vi "Motion Profile Tester.vi"() -> ()   [LabVIEW 2015]
uses:
  <vilib>/Rock Robotics/WPI/CAN/TalonSRX/WPI_CANTalonSRX_APIFeedbackSelect.ctl
  <vilib>/Rock Robotics/WPI/CAN/TalonSRX/WPI_CANTalonSRX_MotionProfileTrajectoryPt.ctl
  <vilib>/Rock Robotics/WPI/CAN/TalonSRX/WPI_CANTalonSRX_APIControlMode.ctl
  <vilib>/Rock Robotics/WPI/MotorControl/WPI_MotorControlOpenCANTalonSRX.vi
panel:
  in  "Finish":bool
  in  "(Native Position units/sec)/(Native units for velocity)":dbl
  in  "Quantity of Points to Load Initially":dbl=126.0
  out "Loaded Trajectory Points":u32
  in  "Slave Motor Inverts":bool[](array[boolean])
  in  "Motor ID":dbl
  in  "Slave Motor IDs":dbl[](array[numeric])
  out "Current State":T1(ring)
  in  "Invert Motor":bool=TRUE
  in  "Execute Motion Profile using only Feedfoward":bool
  in  "Soft Limits (rotations)":T2={"Forward Limit Position"=10000.0, "Reverse Limit Position (should be less than foward limit position)"=-10000.0}
  in  "Reverse Soft Limit Enable":bool
  in  "Forward Soft Limit Enable":bool
  in  "Reverse Feedback Sensor":bool
  in  "Feedback Reference":T3=enum."CTR Magnetic Enc (Absolute)"
  in  "PID Values":T4={"P"=0.21, "I"=0.0021, "D"=3.0, "F"=0.12, "I Zone"=1200.0}
  out "error out":errorcluster
  out "Motor Values while Running Profile":cluster{dbl[], dbl[]}[](graph)
  out "Applied Throttle while Running Profile":cluster{dbl[], dbl[]}(graph)
  in  "Run at 100% Power and Graph":bool
  in  "Abort":bool
  in  "Generate, Load, and Run Profile":bool
  in  "Run Profile":bool
  in  "Load Profile":bool
  in  "Generate Profile and Clear Points":bool
  out "Generated Profile":cluster{dbl[], dbl[]}[](graph)
  in  "Mode":T1(ring)
  in  "Duration MS":dbl=10.0
  in  "Rotations to Travel":dbl
  in  "Max Jerk (rotations/sec^3)":dbl
  in  "Max Acceleration (rotations/sec^2)":dbl
  in  "Max Speed (rotations/sec)":dbl
  # "Basic Motor Configuration Settings"
  # "Motion Profile Settings"
  # "If applied throttle exceeds about .95 consistantly in the execution of the profile either max speed acceleration, or jerk must be lowered (or PIDF should be adjusted). If it goes below .8 except at the very beginning or end either max speed, acceleration, or jerk  could be increased. (These numbers are for profiles which are supposed to be completed as quickly as possible. In contexts where the priority is on other things such as reducing the amount of force or jerk acting on a gearbox other metrics must be used.)"
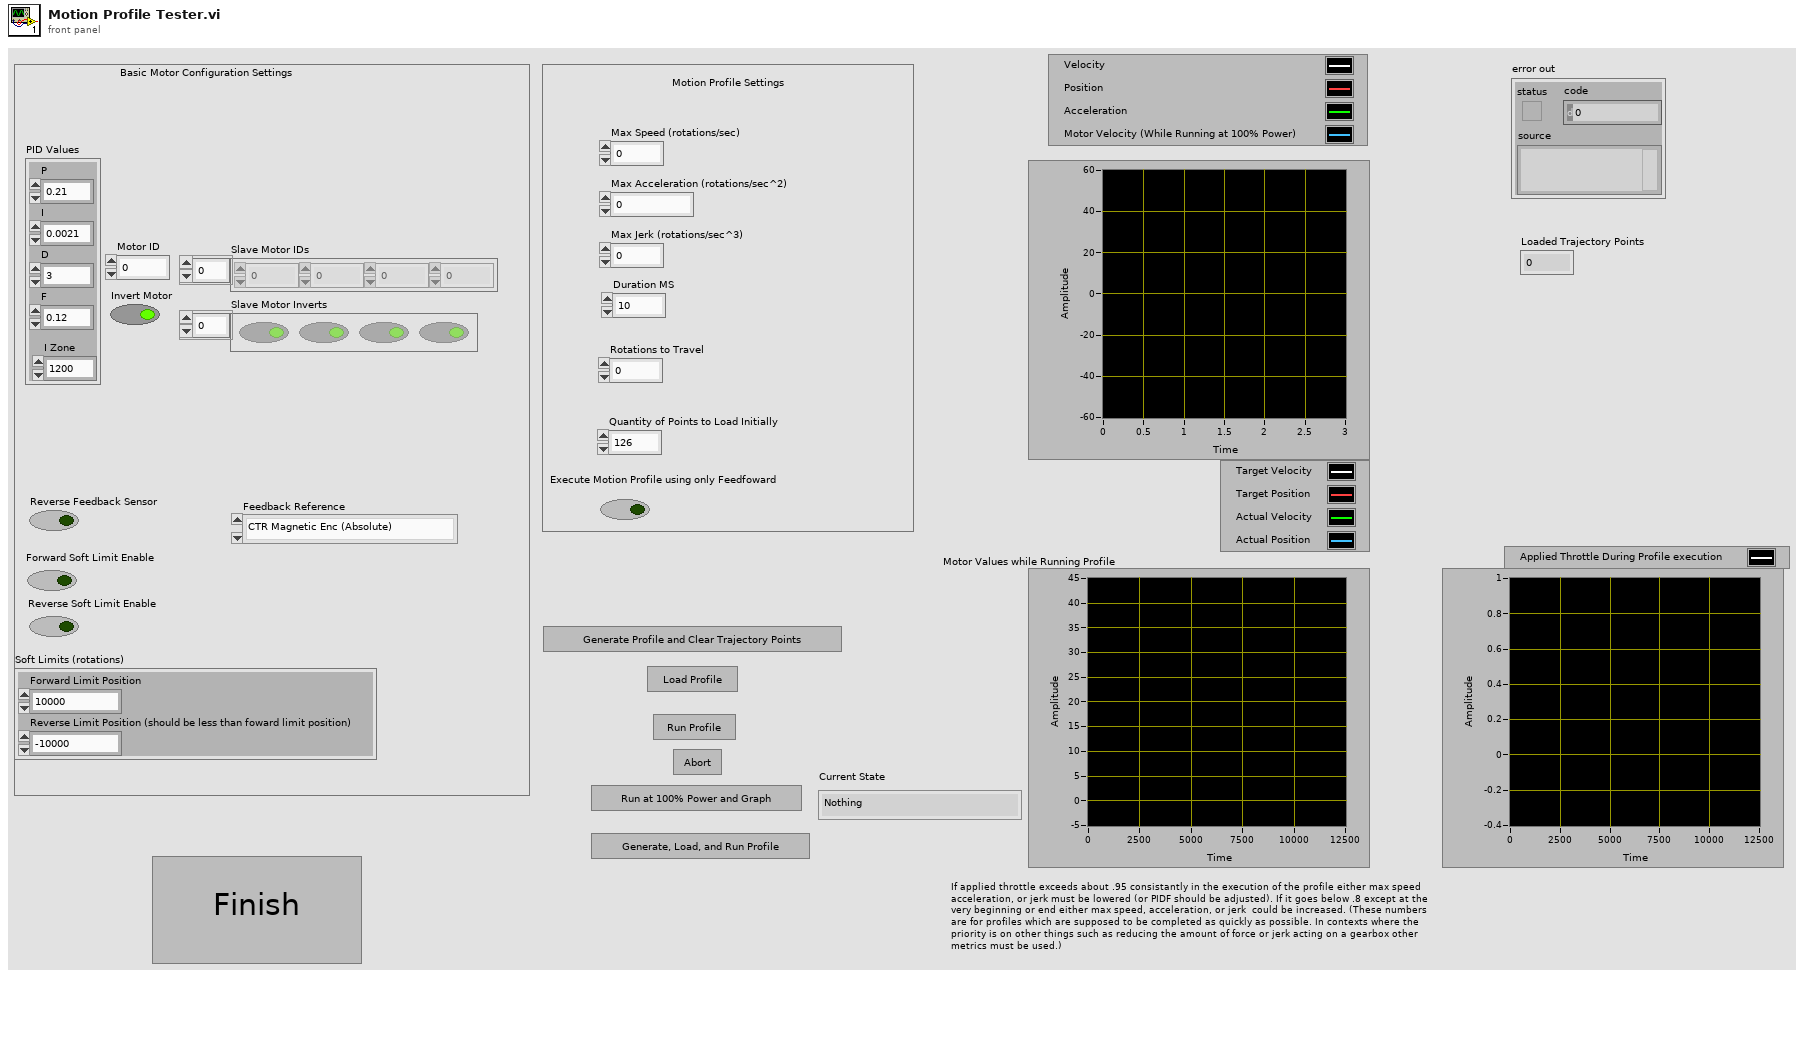
[diagram p1: front panel]
types:
  T1 = enum16{"Nothing", "Generate Profile and Clear", "Load Data to Motor", "Run Profile", "Run at 100% power and log"}
  T2 = cluster{"Forward Limit Position":dbl, "Reverse Limit Position (should be less than foward limit position)":dbl}
  T3 = typedef "WPI_CANTalonSRX_APIFeedbackSelect.ctl" = enum16{"Digital Quadrature Encoder", "Analog Potentiometer", "Analog Encoder", "Count on Quad-A (Rising-Edge)", "Count on Quad-A (Falling-Edge)", "CTR Magnetic Enc (Absolute)", "CTR Magnetic Enc (Relative)", "Pulse Width"}
  T4 = cluster{"P":dbl, "I":dbl, "D":dbl, "F":dbl, "I Zone":dbl}
  T5 = typedef "WPI_CANTalonSRX_APIControlMode.ctl" = enum8{"Percent VBus", "Speed", "Position", "Slave", "Unchanged / Invalid", "Voltage Compensation", "Current", "Motion Profile"}
  T6 = typedef "WPI_MotorControlDeviceRef.ctl" = cluster{"DeviceStatus":errorcluster, "Type":T7, "PWM":cluster{"PWM Channel":T8, "DeadBand":T9}, "CAN":cluster{"Device Number":u8, "Control Mode":T10, "Semaphore":T11, "Max Vout":dbl, "TalonSRX Control Mode":T5}, "Invert":bool}
  T7 = typedef "WPI_MotorControlType.ctl" = enum16{"PWM", "CAN", "CANTalonSRX"}
  T8 = typedef "FPGA_DIOPWMChannel.ctl" = enum8{"PWM 0", "PWM 1", "PWM 2", "PWM 3", "PWM 4", "PWM 5", "PWM 6", "PWM 7", "PWM 8", "PWM 9", "PWM MXP 0", "PWM MXP 1", "PWM MXP 2", "PWM MXP 3", "PWM MXP 4", "PWM MXP 5", "PWM MXP 6", "PWM MXP 7", "PWM MXP 8", "PWM MXP 9", "Invalid"}
  T9 = typedef "WPI_PWMDeadband.ctl" = cluster{"Name":string, "maxPositivePwm":i32, "minPositivePwm":i32, "centerPwm":i32, "maxNegativePwm":i32, "minNegativePwm":i32, "angularRange":u16}
  T10 = typedef "WPI_CANJaguar_ControlMode.ctl" = enum8{"Percent VBus", "Current", "Speed", "Position", "Voltage"}
  T11 = typedef "Semaphore RefNum" = refnum<k1>
  T12 = typedef "WPI_CANTalonSRX_MotionProfileTrajectoryPt.ctl" = cluster{"Duration Ms":u8, "Velocity":dbl, "Position":dbl, "Profile Slot Select":u8, "Is Last":bool, "Velocity Only":bool, "Zero Position":bool, "Compress Code":u8, "Same Velocity":i32, "Delta Position":i32, "Count":u8}
  T13 = enum16{"Nothing", "Generate Profile and Clear", "Load Data to Motor", "Run Profile"}
  T14 = enum16{"Nothing", "Generate Profile and Clear", "Load Data to Motor", "Run Profile", "Run at 100% power and log"}[]
  T15 = typedef "WPI_CANTalonSRX_GlobalStatus.ctl" = cluster{"Applied Throttle":dbl, "Module Enabled":bool, "CAN Error":errorcluster, "Closed Loop Error":dbl, "Forward Limit Switch Closed":bool, "Reverse Limit Switch Closed":bool, "Sensor Position":dbl, "Sensor Velocity":dbl, "Current":dbl, "Sticky Fault - Over Temp":bool, "Sticky Fault - Under Voltage":bool, "Sticky Fault - Forward Limit":bool, "Sticky Fault - Reverse Limit":bool, "Sticky Fault - Forward Soft Limit":bool, "Sticky Fault - Reverse Soft Limit":bool, "Brake is Enabled":bool, "Encoder Position":dbl, "Encoder Velocity":dbl, "Encoder Index Count":dbl, "Encoder A Pin State":bool, "Encoder B Pin State":bool, "Encoder Index Pin State":bool, "Analog In":dbl, "Analog In Velocity":dbl, "Temperature (C)":dbl, "Battery Voltage":dbl, "Control 5 Is Supported":bool, "Current Profile Slot Select":dbl, "Pos Div 8":bool, "Vel Div 4":bool, "Pulse Width Position":i32, "Pulse Width Velocity":i32, "Pulse Width Rise To Rise (us)":i32, "Pulse Width Rise To Fall (us)":i32, "Mot Prof Active Is Under Run":bool, "Mot Prof Active Has Under Run":bool, "Mot Prof Active Is Last":bool, "Mot Prof Active Velocity Only":bool, "Mot Prof Active Is Valid":bool, "Mot Prof Buffer Is Full":bool, "Mot Prof Active Profile Slot Select":i32, "Mot Prof NextID":i32, "Mot Prof Count":i32, "Mot Prof Active Velocity":dbl, "Mot Prof Active Position":dbl, "Mot Prof Output Enable":i32}
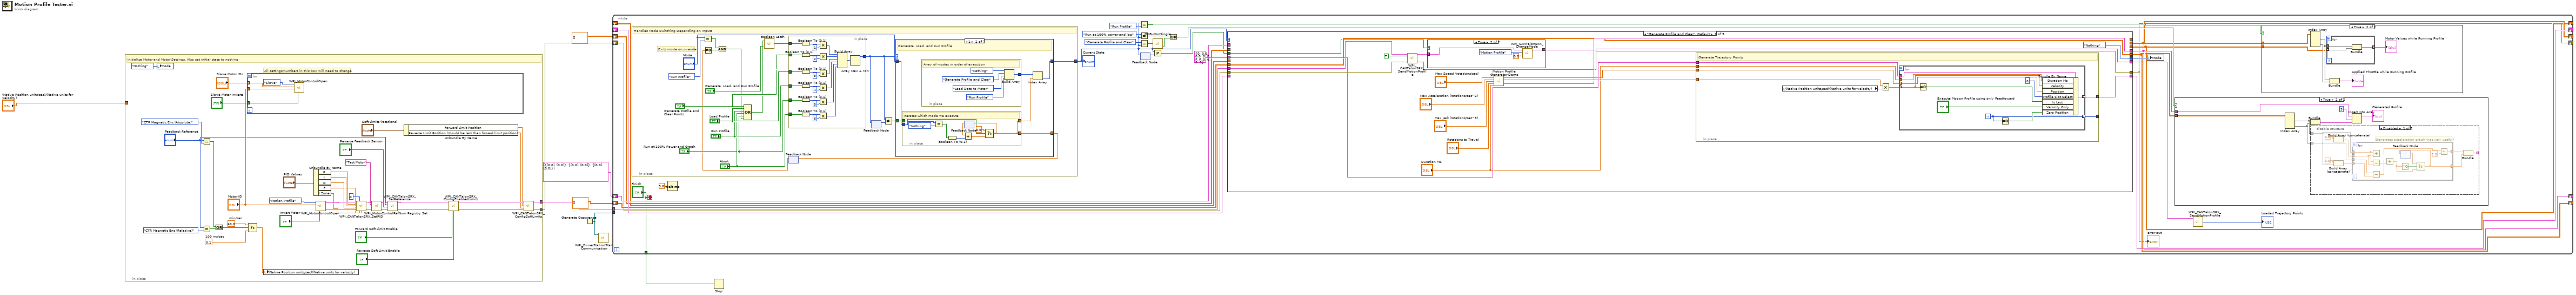
[diagram p0: block diagram]
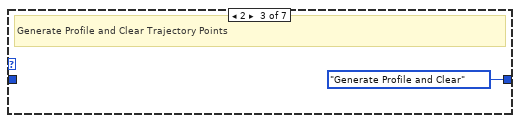
[diagram p6: hidden frame]
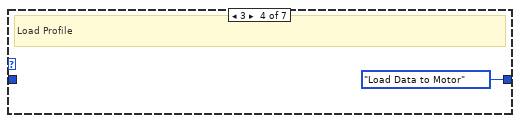
[diagram p7: hidden frame]
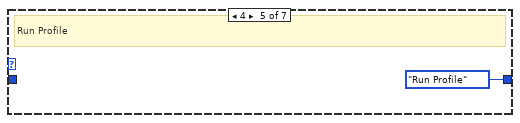
[diagram p8: hidden frame]
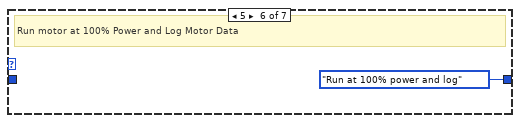
[diagram p9: hidden frame]
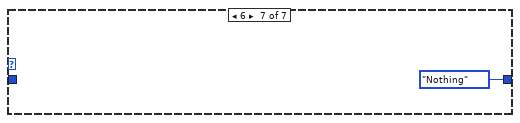
[diagram p10: hidden frame]
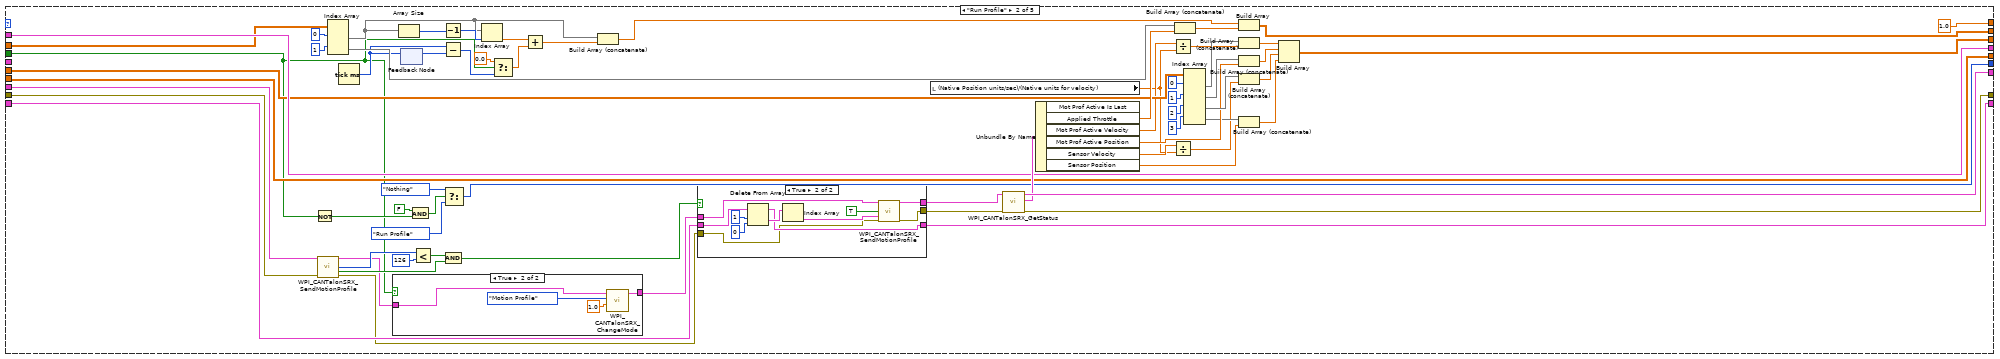
[diagram p12: hidden frame]
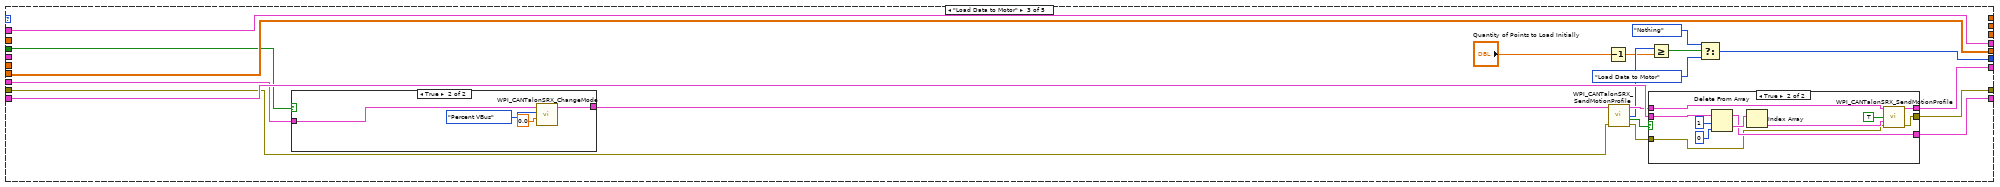
[diagram p15: hidden frame]
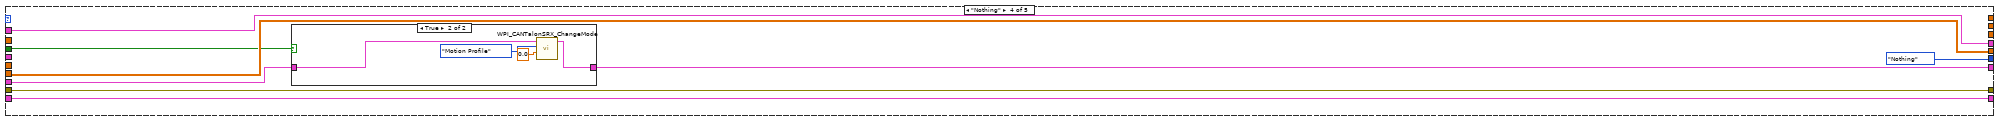
[diagram p18: hidden frame]
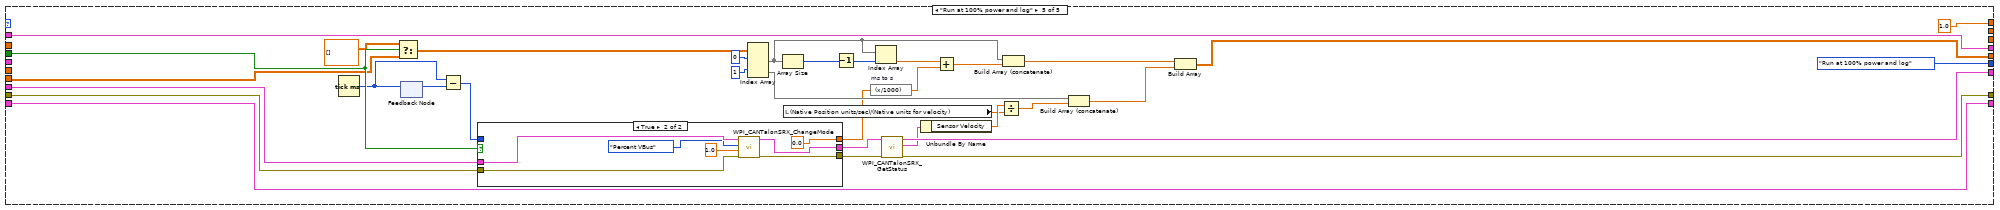
[diagram p20: hidden frame]
diagram:
  n1 = in-place {
    in-place-border: [w45] -> w8
    in-place-border: [w32] -> w4
    in-place-border: "(Native Position units/sec)/(Native units for velocity)" -> [_]
    w10 = 0.1  # 100 ms/sec
    w11 = 60.0  # min/sec
    # "All settings/numbers in this box will need to change"
    # "Initialize Motor and Motor Settings. Also set initial state to nothing"
    n2 = local write "Mode"(T1."Nothing" ("Mode")) -> ()
    n3 = Equal?(x="Feedback Reference", y=WPI_CANTalonSRX_APIFeedbackSelect."CTR Magnetic Enc (Absolute)") -> (x = y?=w16:bool)
    n4 = Equal?(x="Feedback Reference", y=WPI_CANTalonSRX_APIFeedbackSelect."CTR Magnetic Enc (Relative)") -> (x = y?=w13:bool)
    n5 = Or(x=w16, y=w13) -> (x .or. y?=w12:bool)
    n6 = for {
      tunnel: "Motor ID" -> [w53]
      tunnel: "Slave Motor IDs" -> [w52] mode=indexing
      tunnel: "Slave Motor Inverts" -> [w50] mode=indexing
      n7 = call-poly <vilib>:"WPI_MotorControlOpen.vi"("Invert"=w50, "Master Device Number"=w53, "Device Number"=w52, "Control Mode"=WPI_CANTalonSRX_APIControlMode."Slave") -> ()  [unwired: 6 in, 2 out]
    }
    n8 = Select(t=w11, s=w12, f=w10) -> (s? t:f=w9:dbl)
    n9 = local write "(Native Position units/sec)/(Native units for velocity)"(w9) -> ()
    n10 = Unbundle By Name("PID Values") -> ("P"=w25:dbl, "I"=w24:dbl, "D"=w23:dbl, "F"=w22:dbl, "I Zone"=w21:dbl)
    n11 = call-poly <vilib>:"WPI_MotorControlOpen.vi"("Invert"="Invert Motor", "Device Number"="Motor ID", "Control Mode"=WPI_CANTalonSRX_APIControlMode."Motion Profile") -> ("error out"=w47:errorcluster, "MotorControlDeviceRef"=w48:T6)  [unwired: 7 in]
    n12 = call <vilib>:"WPI_CANTalonSRX_SetPID.vi"("CAN Talon SRX Ref"=w48, "Parameter Slot"=u8 0, "P"=w25, "I"=w24, "D"=w23, "error in (no error)"=w47, "F"=w22, "I Zone"=w21) -> ("CAN Talon SRX Ref"=w40:T6, "error out"=w38:errorcluster)  [unwired: 6 in]
    n13 = call <vilib>:"WPI_MotorControlRefNum Registry Set.vi"("error in (no error)"=w38, "refnum name"="Test Motor", "MotorControlDevRef"=w40) -> ("error out"=w37:errorcluster, "MotorControlDevRef"=w39:T6)  [unwired: 7 in]
    n14 = call <vilib>:"WPI_CANTalonSRX_SetReference.vi"("error in (no error)"=w37, "Reverse Feedback Sensor"="Reverse Feedback Sensor", "Feedback Reference"="Feedback Reference", "CAN Talon SRX Ref"=w39) -> ("error out"=w34:errorcluster, "CAN Talon SRX Ref"=w35:T6)  [unwired: 6 in]
    n15 = Unbundle By Name("Soft Limits (rotations)") -> ("Forward Limit Position"=w28:dbl, "Reverse Limit Position (should be less than foward limit position)"=w27:dbl)
    n16 = call <vilib>:"WPI_CANTalonSRX_ConfigEnabledLimits.vi"("CAN Talon SRX Ref"=w35, "error in (no error)"=w34, "Forward Soft Limit Enable"="Forward Soft Limit Enable", "Reverse Soft Limit Enable"="Reverse Soft Limit Enable") -> ("CAN Talon SRX Ref"=w43:T6, "error out"=w44:errorcluster)  [unwired: 10 in]
    n17 = call <vilib>:"WPI_CANTalonSRX_ConfigSoftLimits.vi"("CAN Talon SRX Ref"=w43, "Forward Limit Position"=w28, "Reverse Limit Position"=w27, "error in (no error)"=w44) -> ("CAN Talon SRX Ref"=w45:T6, "error out"=w32:errorcluster)  [unwired: 10 in]
  }
  n18 = Generate Occurrence() -> (w3:refnum<k4>)
  n19 = call <vilib>:"WPI_DriverStationStart Communication.vi"("occurrence"=w3) -> ()  [unwired: 11 in]
  n20 = while {
    tunnel: w8 -> [w83]
    shift-right: [w81] -> _
    shift-left: _ -> [w79]
    shift-right: [w73] -> _
    shift-left: cluster{dbl[], dbl[]}[] [{[0.0], [0.0]}, {[0.0], [0.0]}, {[0.0], [0.0]}] ("XY Graph") -> [w75]
    shift-right: [w72] -> _
    shift-left: dbl[][] [] -> [w74]
    shift-right: [w64] -> _
    shift-left: dbl[][] [] -> [w67]
    shift-right: [w62] -> _
    shift-left: _ -> [w63]
    shift-right: [w57] -> _
    shift-left: w4 -> [w58]
    tunnel: w3 -> [_]
    tunnel: ["Finish"] -> w1
    stop <- "Finish" stop-if-true
    n21 = in-place {
      in-place-border: [w139] -> w61
      # "Exits mode on overide"
      # "Handles Mode Switching Depending on Inputs"
      n22 = Equal?(x="Mode", y=T13."Run Profile") -> (x = y?=w132:bool)
      n23 = feedback #1() -> (w123:dbl)  [unwired: 1 in]
      n24 = Not Equal To 0?(x=w123) -> (x != 0?=w122:bool)
      n25 = And(x=w132, y=w122) -> (x .and. y?=w125:bool)
      n26 = Compound Arithmetic op=OR("Generate Profile and Clear Points", "Load Profile", "Run Profile", "Abort", "Run at 100% Power and Graph", w125) -> (w131:bool)
      n27 = call "Boolean Latch.vi"("Input"="Generate, Load, and Run Profile", "Reset"=w131) -> ("Output"=w130:bool)
      n28 = in-place {
        in-place-border: "Generate Profile and Clear Points" -> [w166]
        in-place-border: "Load Profile" -> [w161]
        in-place-border: w130 -> [w159]
        in-place-border: "Run Profile" -> [w157]
        in-place-border: [w155] -> w128
        in-place-border: "Abort" -> [w146]
        in-place-border: "Run at 100% Power and Graph" -> [w143]
        n29 = Boolean To (0,1)(Boolean=w159) -> (0, 1=w153:i16)
        n30 = Boolean To (0,1)(Boolean=w166) -> (0, 1=w165:i16)
        n31 = Boolean To (0,1)(Boolean=w161) -> (0, 1=w163:i16)
        n32 = Boolean To (0,1)(Boolean=w157) -> (0, 1=w154:i16)
        n33 = Boolean To (0,1)(Boolean=w143) -> (0, 1=w142:i16)
        n34 = Boolean To (0,1)(Boolean=w146) -> (0, 1=w145:i16)
        n35 = Multiply(x=w153, y=i16 1) -> (x*y=w150:i16)
        n36 = Multiply(x=w165, y=i16 2) -> (x*y=w149:i16)
        n37 = Multiply(x=w163, y=i16 3) -> (x*y=w148:i16)
        n38 = Multiply(x=w154, y=i16 4) -> (x*y=w147:i16)
        n39 = Multiply(x=w142, y=i16 5) -> (x*y=w141:i16)
        n40 = Multiply(x=w145, y=i16 6) -> (x*y=w144:i16)
        n41 = Build Array(w150, w149, w148, w147, w141, w144) -> (w156:i16[])
        n42 = Array Max & Min(array=w156) -> (max value=w155:i16)  [unwired: 3 out]
      }
      n43 = feedback-in #2(w128) -> ()
      n44 = feedback #2() -> (w127:i16)  [unwired: 1 in]
      n45 = Not Equal?(x=w128, y=w127) -> (x != y?=w126:bool)
      n46 = case shown="1" w128 {
        tunnel: [w167 w170 T1."Generate Profile and Clear" ("Mode") T1."Load Data to Motor" ("Mode") T1."Run Profile" ("Mode") T1."Run at 100% power and log" ("Mode") T1."Nothing" ("Mode")] -> w139
        tunnel: "Mode" -> [w167 w173 _ _ _ _ _]
        tunnel: w126 -> [_ w169 _ _ _ _ _]
        tunnel: [_ w168 _ _ _ _ _] -> w124
        frame 0, Default {
          # "Carry last operation"
        }
        frame 1 {
          # "Generate, Load, and Run Profile"
          n47 = in-place {
            in-place-border: w173 -> [w182]
            in-place-border: w169 -> [w175]
            in-place-border: [w174] -> w171
            in-place-border: [w174] -> w168
            # "Iterates which mode we execute"
            n48 = Equal?(x=w182, y=T1."Nothing") -> (x = y?=w181:bool)
            n49 = Boolean To (0,1)(Boolean=w181) -> (0, 1=w180:i16)
            n50 = feedback #3() -> (w179:dbl)  [unwired: 1 in]
            n51 = Add(x=w179, y=w180) -> (x+y=w177:dbl)
            n52 = Select(t=0.0, s=w175, f=w177) -> (s? t:f=w174:dbl)
            n53 = feedback-in #3(w174) -> ()
          }
          n54 = in-place {
            in-place-border: [w187] -> w172
            # "Array of modes in order of execution"
            n55 = Build Array(T1."Nothing" ("Mode"), T1."Generate Profile and Clear" ("Mode"), T1."Load Data to Motor" ("Mode"), T1."Run Profile" ("Mode")) -> (w187:T14)
          }
          n56 = Index Array(array=w172, index=w171) -> (element=w170:T1)
        }
        frame 2 {
          # "Generate Profile and Clear Trajectory Points"
        }
        frame 3 {
          # "Load Profile"
        }
        frame 4 {
          # "Run Profile"
        }
        frame 5 {
          # "Run motor at 100% Power and Log Motor Data"
        }
        frame 6 {
        }
      }
      n57 = feedback-in #1(w124) -> ()
    }
    "Current State" <- w61
    n58 = Wait (ms)(milliseconds to wait=3.0) -> ()  [unwired: 1 out]
    n59 = Equal?(x=w61, y=T1."Run Profile") -> (x = y?=w65:bool)
    n60 = Equal?(x=T1."Run at 100% power and log", y=w61) -> (x = y?=w68:bool)
    n61 = Equal?(x=T1."Generate Profile and Clear", y=w61) -> (x = y?=w71:bool)
    n62 = feedback-in #4(w61) -> ()
    n63 = feedback #4() -> (w60:T1)  [unwired: 1 in]
    n64 = Not Equal?(x=w61, y=w60) -> (x != y?=w59:bool)
    n65 = call "OnButtonSingle.vi"("Input"=w71) -> ("Released"=w70:bool)  [unwired: 1 out]
    n66 = Or(x=w68, y=w70) -> (x .or. y?=w69:bool)
    n67 = case shown="\"Generate Profile and Clear\", Default" w61 {
      tunnel: w83 -> [w207 w299 w324 w361 w405]
      tunnel: T12 {"Duration Ms"=0, "Velocity"=0.0, "Position"=0.0, "Profile Slot Select"=0, "Is Last"=FALSE, "Velocity Only"=FALSE, "Zero Position"=FALSE, "Compress Code"=0, "Same Velocity"=0, "Delta Position"=0, "Count"=0} ("New Point") -> [w206 _ _ _ _]
      tunnel: [w203 w249 w337 w366 w379] -> w81
      tunnel: [T1."Nothing" ("Mode") w296 w335 T1."Nothing" ("Mode") T1."Run at 100% power and log" ("Mode")] -> w80
      tunnel: w79 -> [_ w250 w339 w366 w379]
      tunnel: [w193 w298 w334 w359 w401] -> w56
      tunnel: [_ 1.0 _ _ 1.0] -> _
      tunnel: w59 -> [w195 w239 w322 w360 w393]
      tunnel: [w200 w292 w330 w363 w394] -> w72
      tunnel: [w201 w293 w331 w364 w400] -> w73
      tunnel: w75 -> [_ w293 w331 w364 w400]
      tunnel: w74 -> [w200 w292 w330 w363 w392]
      tunnel: w67 -> [_ w244 _ _ _]
      tunnel: [_ w288 _ _ _] -> w64
      tunnel: w63 -> [_ w281 _ _ _]
      tunnel: [_ w268 _ _ _] -> w62
      tunnel: w58 -> [w197 w248 w327 w362 w378]
      tunnel: [w196 w245 w325 w362 w376] -> w57
      frame "Generate Profile and Clear", Default {
        n68 = call <vilib>:"WPI_CANTalonSRX_SendMotionProfile.vi"("CAN Talon SRX Ref"=w207, "Clear"=TRUE, "error in"=w197) -> ("CAN Talon SRX Ref Out"=w194:T6, "error out"=w196:errorcluster)  [unwired: 9 in, 2 out]
        n69 = case shown="True" w195 {
          tunnel: w194 -> [w212 w214]
          tunnel: [w212 w216] -> w193
          frame False {
          }
          frame True {
            n70 = call <vilib>:"WPI_CANTalonSRX_ChangeMode.vi"("Output"=0.0, "Control Mode"=WPI_CANTalonSRX_APIControlMode."Motion Profile", "CAN Talon SRX Ref"=w214) -> ("CAN Talon SRX Ref"=w216:T6)  [unwired: 7 in, 1 out]
          }
        }
        n71 = call "Motion Profile Generator-Demo.vi"("Max Speed (rotations/sec)"="Max Speed (rotations/sec)", "Max Acceleration (rotations/sec^2)"="Max Acceleration (rotations/sec^2)", "Max Jerk (rotations/sec^3)"="Max Jerk (rotations/sec^3)", "Rotations to Travel"="Rotations to Travel", "Duration MS"="Duration MS") -> ("Position rotations"=w204:dbl[], "velocity rotations/sec"=w205:dbl[], "XY Graph"=w201:cluster{dbl[], dbl[]}[])  [unwired: 7 in, 1 out]
        n72 = in-place {
          in-place-border: w206 -> [w224]
          in-place-border: w205 -> [w219]
          in-place-border: w204 -> [w223]
          in-place-border: "Duration MS" -> [w222]
          in-place-border: [w221] -> w203
          in-place-border: [w220] -> _
          # "Generate Trajectory Points"
          n73 = local read "(Native Position units/sec)/(Native units for velocity)"() -> (w217:dbl)
          n74 = Multiply(x=w219, y=w217) -> (x*y=w218:dbl[])
          n75 = for {
            tunnel: w224 -> [w234]
            tunnel: w218 -> [w230] mode=indexing
            tunnel: w223 -> [w232] mode=indexing
            tunnel: w222 -> [w231]
            tunnel: [w226] -> w221 mode=indexing
            tunnel: [w225] -> w220 mode=indexing
            i -> [w225]
            n76 = Equal To 0?(x=w230) -> (x = 0?=w229:bool)
            n77 = Equal To 0?(x=w225) -> (x = 0?=w227:bool)
            n78 = Bundle By Name(cluster=w234, "Duration Ms"=w231, "Velocity"=w230, "Position"=w232, "Profile Slot Select"=u8 0, "Is Last"=w229, "Velocity Only"="Execute Motion Profile using only Feedfoward", "Zero Position"=w227) -> (w226:T12)
          }
        }
      }
      frame "Run Profile" {
        n79 = Not(x=w239) -> (.not. x?=w240:bool)
        n80 = call <vilib>:"WPI_CANTalonSRX_SendMotionProfile.vi"("CAN Talon SRX Ref"=w299, "error in"=w248) -> ("CAN Talon SRX Ref Out"=w243:T6, "Count"=w256:u32, "Ready For Next"=w253:bool, "error out"=w247:errorcluster)  [unwired: 10 in]
        n81 = Index Array(array=w244, index (row) #1=0 ("index (row)"), index (row) #2=1 ("index (row)")) -> (element #1=w261:dbl[], element #2=w290:dbl[])  [unwired: 2 in]
        n82 = Tick Count (ms)() -> (millisecond timer value=w267:u32)
        n83 = case shown="True" w239 {
          tunnel: w243 -> [w301 w303]
          tunnel: [w301 w305] -> w242
          frame False {
          }
          frame True {
            n84 = call <vilib>:"WPI_CANTalonSRX_ChangeMode.vi"("Output"=1.0, "Control Mode"=WPI_CANTalonSRX_APIControlMode."Motion Profile", "CAN Talon SRX Ref"=w303) -> ("CAN Talon SRX Ref"=w305:T6)  [unwired: 7 in, 1 out]
          }
        }
        n85 = Array Size(array=w261) -> (size(s)=w263:i32)
        n86 = feedback #5() -> (w266:u32)  [unwired: 1 in]
        n87 = feedback-in #5(w267) -> ()
        n88 = And(x=FALSE, y=w240) -> (x .and. y?=w241:bool)
        n89 = Less?(x=w256, y=u32 126) -> (x < y?=w254:bool)
        n90 = Subtract(x=w267, y=w266) -> (x-y=w264:u32)
        n91 = Decrement(x=w263) -> (x-1=w262:i32)
        n92 = And(x=w254, y=w253) -> (x .and. y?=w252:bool)
        n93 = Select(t=T1."Nothing" ("Mode"), s=w241, f=T1."Run Profile" ("Mode")) -> (s? t:f=w296:T1)
        n94 = Index Array(array=w261, index=w262) -> (element=w260:dbl)
        n95 = Select(t=0.0, s=w239, f=w264) -> (s? t:f=w259:dbl)
        n96 = Add(x=w260, y=w259) -> (x+y=w289:dbl)
        n97 = Build Array (concatenate)(w261, w289) -> (w287:dbl[])
        n98 = case shown="True" w252 {
          tunnel: w250 -> [w308 w319]
          tunnel: w242 -> [w307 w316]
          tunnel: [w308 w315] -> w249
          tunnel: [w307 w314] -> w251
          tunnel: w247 -> [w306 w310]
          tunnel: [w306 w309] -> w246
          frame False {
          }
          frame True {
            n99 = Delete From Array(array=w319, length=1, index=0) -> (deleted portion=w317:T12[], array with subset deleted=w315:T12[])
            n100 = Index Array(array=w317) -> (element=w311:T12)  [unwired: 1 in]
            n101 = call <vilib>:"WPI_CANTalonSRX_SendMotionProfile.vi"("CAN Talon SRX Ref"=w316, "Push"=TRUE, "New Point"=w311, "error in"=w310) -> ("CAN Talon SRX Ref Out"=w314:T6, "error out"=w309:errorcluster)  [unwired: 8 in, 2 out]
          }
        }
        n102 = local read "(Native Position units/sec)/(Native units for velocity)"() -> (w235:dbl)
        n103 = call <vilib>:"WPI_CANTalonSRX_GetStatus.vi"("error in (no error)"=w246, "CAN Talon SRX Ref"=w251) -> ("error out"=w245:errorcluster, "Talon SRX Status"=w297:T15, "CAN Talon SRX Ref"=w298:T6)  [unwired: 7 in]
        n104 = Unbundle By Name(w297) -> ("Applied Throttle"=w291:dbl, "Mot Prof Active Velocity"=w258:dbl, "Mot Prof Active Position"=w274:dbl, "Sensor Velocity"=w237:dbl, "Sensor Position"=w272:dbl)  [unwired: 1 out]
        n105 = Divide(x=w258, y=w235) -> (x/y=w257:dbl)
        n106 = Divide(x=w237, y=w235) -> (x/y=w236:dbl)
        n107 = Build Array (concatenate)(w290, w291) -> (w286:dbl[])
        n108 = Index Array(array=w281, index (row) #1=0 ("index (row)"), index (row) #2=1 ("index (row)"), index (row) #3=2 ("index (row)"), index (row) #4=3 ("index (row)")) -> (element #1=w284:dbl[], element #2=w285:dbl[], element #3=w275:dbl[], element #4=w270:dbl[])  [unwired: 4 in]
        n109 = Build Array(w287, w286) -> (w288:dbl[][])
        n110 = Build Array (concatenate)(w284, w257) -> (w283:dbl[])
        n111 = Build Array (concatenate)(w285, w274) -> (w282:dbl[])
        n112 = Build Array (concatenate)(w275, w236) -> (w273:dbl[])
        n113 = Build Array (concatenate)(w270, w272) -> (w269:dbl[])
        n114 = Build Array(w283, w282, w273, w269) -> (w268:dbl[][])
      }
      frame "Load Data to Motor" {
        n115 = case shown="True" w322 {
          tunnel: w324 -> [w340 w344]
          tunnel: [w340 w343] -> w323
          frame False {
          }
          frame True {
            n116 = call <vilib>:"WPI_CANTalonSRX_ChangeMode.vi"("Output"=0.0, "Control Mode"=WPI_CANTalonSRX_APIControlMode."Percent VBus", "CAN Talon SRX Ref"=w344) -> ("CAN Talon SRX Ref"=w343:T6)  [unwired: 7 in, 1 out]
          }
        }
        n117 = Decrement(x="Quantity of Points to Load Initially") -> (x-1=w320:dbl)
        n118 = call <vilib>:"WPI_CANTalonSRX_SendMotionProfile.vi"("CAN Talon SRX Ref"=w323, "error in"=w327) -> ("CAN Talon SRX Ref Out"=w338:T6, "Count"=w328:u32, "Ready For Next"=w336:bool, "error out"=w326:errorcluster)  [unwired: 10 in]
        n119 = case shown="True" w336 {
          tunnel: w339 -> [w347 w358]
          tunnel: w338 -> [w346 w355]
          tunnel: [w347 w354] -> w337
          tunnel: [w346 w353] -> w334
          tunnel: w326 -> [w345 w349]
          tunnel: [w345 w348] -> w325
          frame False {
          }
          frame True {
            n120 = Delete From Array(array=w358, length=1, index=0) -> (deleted portion=w356:T12[], array with subset deleted=w354:T12[])
            n121 = Index Array(array=w356) -> (element=w350:T12)  [unwired: 1 in]
            n122 = call <vilib>:"WPI_CANTalonSRX_SendMotionProfile.vi"("CAN Talon SRX Ref"=w355, "Push"=TRUE, "New Point"=w350, "error in"=w349) -> ("CAN Talon SRX Ref Out"=w353:T6, "error out"=w348:errorcluster)  [unwired: 8 in, 2 out]
          }
        }
        n123 = Greater Or Equal?(x=w328, y=w320) -> (x >= y?=w329:bool)
        n124 = Select(t=T1."Nothing" ("Mode"), s=w329, f=T1."Load Data to Motor" ("Mode")) -> (s? t:f=w335:T1)
      }
      frame "Nothing" {
        n125 = case shown="True" w360 {
          tunnel: w361 -> [w367 w371]
          tunnel: [w367 w370] -> w359
          frame False {
          }
          frame True {
            n126 = call <vilib>:"WPI_CANTalonSRX_ChangeMode.vi"("Output"=0.0, "Control Mode"=WPI_CANTalonSRX_APIControlMode."Motion Profile", "CAN Talon SRX Ref"=w371) -> ("CAN Talon SRX Ref"=w370:T6)  [unwired: 7 in, 1 out]
          }
        }
      }
      frame "Run at 100% power and log" {
        n127 = Tick Count (ms)() -> (millisecond timer value=w383:u32)
        n128 = Select(t=dbl[][] [], s=w393, f=w392) -> (s? t:f=w390:dbl[][])
        n129 = feedback #6() -> (w382:u32)  [unwired: 1 in]
        n130 = feedback-in #6(w383) -> ()
        n131 = Subtract(x=w383, y=w382) -> (x-y=w381:u32)
        n132 = case shown="True" w393 {
          tunnel: w405 -> [w408 w415]
          tunnel: [w408 w414] -> w402
          tunnel: [w407 0.0] -> w375
          tunnel: w381 -> [w407 _]
          tunnel: w378 -> [w406 w412]
          tunnel: [w406 w411] -> w377
          frame False {
          }
          frame True {
            n133 = call <vilib>:"WPI_CANTalonSRX_ChangeMode.vi"("error in (no error)"=w412, "Output"=1.0, "Control Mode"=WPI_CANTalonSRX_APIControlMode."Percent VBus", "CAN Talon SRX Ref"=w415) -> ("error out"=w411:errorcluster, "CAN Talon SRX Ref"=w414:T6)  [unwired: 6 in]
          }
        }
        n134 = Index Array(array=w390, index (row) #1=0 ("index (row)"), index (row) #2=1 ("index (row)")) -> (element #1=w386:dbl[], element #2=w397:dbl[])  [unwired: 2 in]
        n135 = Array Size(array=w386) -> (size(s)=w387:i32)
        n136 = local read "(Native Position units/sec)/(Native units for velocity)"() -> (w372:dbl)
        n137 = Decrement(x=w387) -> (x-1=w385:i32)
        n138 = expression code="(x/1000)" "ms to s"(w375) -> (w389:dbl)
        n139 = Index Array(array=w386, index=w385) -> (element=w384:dbl)
        n140 = call <vilib>:"WPI_CANTalonSRX_GetStatus.vi"("error in (no error)"=w377, "CAN Talon SRX Ref"=w402) -> ("error out"=w376:errorcluster, "Talon SRX Status"=w380:T15, "CAN Talon SRX Ref"=w401:T6)  [unwired: 7 in]
        n141 = Unbundle By Name(w380) -> ("Sensor Velocity"=w374:dbl)
        n142 = Add(x=w384, y=w389) -> (x+y=w388:dbl)
        n143 = Divide(x=w374, y=w372) -> (x/y=w373:dbl)
        n144 = Build Array (concatenate)(w386, w388) -> (w396:dbl[])
        n145 = Build Array (concatenate)(w397, w373) -> (w395:dbl[])
        n146 = Build Array(w396, w395) -> (w394:dbl[][])
      }
    }
    "error out" <- w57
    n147 = local write "Mode"(w80) -> ()
    n148 = case shown="True" w69 {
      tunnel: w73 -> [_ w99]
      tunnel: w72 -> [_ w96]
      frame False {
      }
      frame True {
        n149 = Index Array(array=w96) -> (element #1=w94:dbl[], element #2=w93:dbl[])  [unwired: 4 in]
        n150 = Bundle(w94, w93) -> (w95:cluster{dbl[], dbl[]})  [unwired: 1 in]
        n151 = disable-structure shown="Disabled" {
          disable-tunnel: w94 -> [w108 _]
          disable-tunnel: w93 -> [w104 _]
          disable-tunnel: [w100 _] -> _
          frame Disabled {
            # "Generates acceleration graph (not very useful)"
            n152 = Build Array (concatenate)(0.0, w108) -> (w106:dbl[])
            n153 = Build Array (concatenate)(0.0, w104) -> (w103:dbl[])
            n154 = for {
              tunnel: w108 -> [w117] mode=indexing
              tunnel: w106 -> [w116] mode=indexing
              tunnel: w104 -> [w120] mode=indexing
              tunnel: w103 -> [w119] mode=indexing
              tunnel: [w109] -> w102 mode=indexing
              tunnel: [w113] -> w101 mode=indexing
              n155 = Add(x=w117, y=w116) -> (x+y=w115:dbl)
              n156 = Subtract(x=w117, y=w116) -> (x-y=w121:dbl)
              n157 = Subtract(x=w120, y=w119) -> (x-y=w118:dbl)
              n158 = Divide(x=w118, y=w121) -> (x/y=w110:dbl)
              n159 = Equal To 0?(x=w110) -> (x = 0?=w112:bool)
              n160 = feedback #7() -> (w111:dbl)  [unwired: 1 in]
              n161 = Select(t=w111, s=w112, f=w110) -> (s? t:f=w109:dbl)
              n162 = feedback-in #7(w109) -> ()
              n163 = Divide(x=w115, y=2.0) -> (x/y=w113:dbl)
            }
            n164 = Bundle(w101, w102) -> (w100:cluster{dbl[], dbl[]})  [unwired: 1 in]
          }
          frame Enabled {
          }
        }
        n165 = Insert Into Array(array=w99, index=3, new element=w95) -> (→"Generated Profile":cluster{dbl[], dbl[]}[])
      }
    }
    n166 = call <vilib>:"WPI_CANTalonSRX_SendMotionProfile.vi"("CAN Talon SRX Ref"=w56) -> ("Count"=→"Loaded Trajectory Points":u32)  [unwired: 11 in, 3 out]
    n167 = case shown="True" w65 {
      tunnel: w64 -> [_ w89]
      tunnel: w62 -> [_ w84]
      frame False {
      }
      frame True {
        n168 = Index Array(array=w89) -> (element #1=w85:dbl[], element #2=w88:dbl[])  [unwired: 4 in]
        n169 = for {
          tunnel: w85 -> [w92]
          tunnel: w84 -> [w91] mode=indexing
          tunnel: [w90] -> w86 mode=indexing
          n170 = Bundle(w92, w91) -> (w90:cluster{dbl[], dbl[]})  [unwired: 1 in]
        }
        "Motor Values while Running Profile" <- w86
        n171 = Bundle(w85, w88) -> (→"Applied Throttle while Running Profile":cluster{dbl[], dbl[]})  [unwired: 1 in]
      }
    }
  }
  n172 = Stop(stop? (T)=w1) -> ()
